vi "Dispose Lock.vi"(8 "error in (no error)":errorcluster, 11 "Pointer in":refnum<class "Pointer.lvclass">) -> (0 "error out":errorcluster, 3 "Pointer out":refnum<class "Pointer.lvclass">)   [LabVIEW 2016, in "Memory Manager.lvlib" / "Pointer.lvclass"]
uses:
  Pointer.lvclass
  Pointer.lvclass/Pointer.ctl
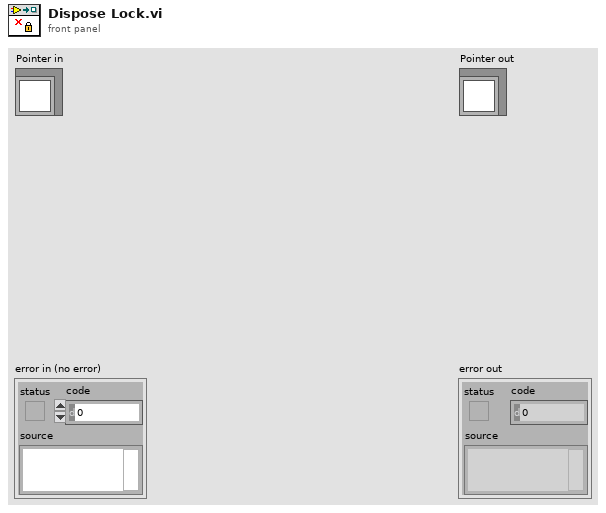
[diagram p1: front panel]
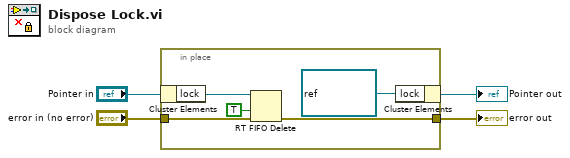
[diagram p0: block diagram]
diagram:
  n1 = in-place {
    in-place-border: "error in (no error)" -> [w8]
    in-place-border: [w6] -> w3
    n2 = in-place-cluster #1("Pointer in") -> ("lock"=w9:refnum<k33>)
    n3 = RT FIFO Delete(0:w9, 2:TRUE ("force destroy? (F)"), 3:w8) -> (11:w6:errorcluster)
    n4 = in-place-cluster #1("lock"=refnum<k33> refnum) -> (→"Pointer out":refnum<class "Pointer.lvclass">)
  }
  "error out" <- w3
